vi ".NET Object Stream Writer.vi"(8 "error in (no error)":errorcluster, 9 "G Object":variant, 11 "TwinCAT ADS in":refnum<class "TwinCAT ADS.lvclass">) -> (0 "error out":errorcluster, 1 ".NET Object Stream":refnum<k24>[](array[refnum]), 2 ".NET Type Stream":refnum<k24>[](array[refnum]), 3 "TwinCAT ADS out":refnum<class "TwinCAT ADS.lvclass">)   [LabVIEW 2018, in "TwinCAT ADS.lvclass"]
uses:
  TwinCAT ADS.lvclass
  <vilib>/Utility/Data Type/NI_Data Type.lvlib
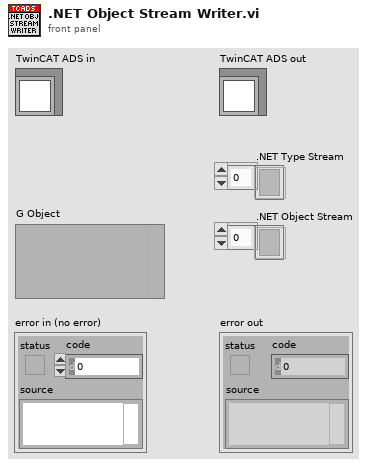
[diagram p1: front panel]
types:
  T1 = typedef "NI_Data Type.lvlib/Data Type.ctl" = enum8{"Invalid Type", "Void", "I8", "I16", "I32", "I64", "U8", "U16", "U32", "U64", "Single Float", "Double Float", "Extended Float", "Single Complex", "Double Complex", "Extended Complex", "Enum U8", "Enum U16", "Enum U32", "Enum U64", "Single Float With Unit", "Double Float With Unit", "Extended Float With Unit", "Single Complex with Unit", "Double Complex with Unit", "Extended Complex with Unit", "Boolean", "String", "Path", "Picture", "Tag", "Array", "Cluster", "Variant", "LV Variant", "Waveform", "Timestamp", "Digital Waveform", "Digital Data", "ExpressData", "Refnum", "External Data", "VI", "Poly VI", "LabVIEW Class Instance", "Fixed Point"}
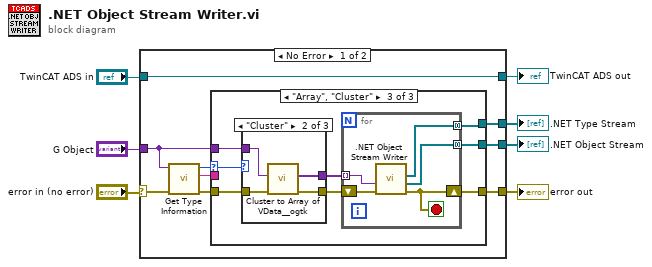
[diagram p0: block diagram]
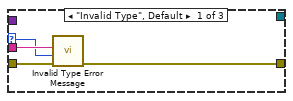
[diagram p2: hidden frame]
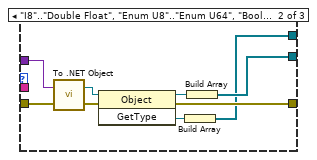
[diagram p3: hidden frame]
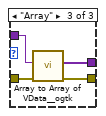
[diagram p5: hidden frame]
diagram:
  n1 = case shown="No Error" "error in (no error)" {
    selector: "error in (no error)" -> [w16 w53]
    tunnel: [w11 w53] -> w2
    tunnel: [w10 w52] -> w5
    tunnel: "TwinCAT ADS in" -> [w10 w52]
    tunnel: "G Object" -> [w14 _]
    tunnel: [w9 _] -> w3
    tunnel: [w8 _] -> w4
    frame No Error {
      n2 = call <vilib>:"Get Type Information.vi"("error in (no error)"=w16, "Variant"=w14) -> ("error out"=w13:errorcluster, "Name"=w12:string, "Type"=w15:T1)  [unwired: 5 in, 2 out]
      n3 = case shown="\"Array\", \"Cluster\"" w15 {
        selector: w15 -> [w18 _ w33]
        tunnel: w14 -> [_ w25 w36]
        tunnel: w13 -> [w20 w27 w37]
        tunnel: w12 -> [w19 _ _]
        tunnel: [w17 w26 w32] -> w11
        tunnel: [_ w23 w30] -> w9
        tunnel: [_ w21 w31] -> w8
        frame "Invalid Type", Default {
          n4 = call "Invalid Type Error Message.vi"("error in (no error)"=w20, "Type"=w18, "Name"=w19) -> ("error out"=w17:errorcluster)  [unwired: 7 in, 1 out]
        }
        frame "I8".."Double Float", "Enum U8".."Enum U64", "Boolean", "String" {
          n5 = call <vilib>:"To .NET Object.vi"("error in (no error)"=w27, "anything"=w25) -> ("error out"=w29:errorcluster, ".NET object"=w28:refnum<k24>)
          n6 = invoke class="Object" method="GetType"(reference=w28, error in=w29) -> (reference out=w24:refnum<k24>, error out=w26:errorcluster, "GetType"=w22:refnum<k24>)  [unwired: 1 in]
          n7 = Build Array(w22) -> (w21:refnum<k24>[])
          n8 = Build Array(w24) -> (w23:refnum<k24>[])
        }
        frame "Array", "Cluster" {
          n9 = case shown="\"Cluster\"" w33 {
            tunnel: w37 -> [w38 w42 w46]
            tunnel: w36 -> [_ w41 w44]
            tunnel: [w38 w40 w45] -> w35
            tunnel: [_ w39 w43] -> w34
            frame "Invalid Type", Default {
            }
            frame "Cluster" {
              n10 = call <userlib>:"Cluster to Array of VData__ogtk.vi"("error in (no error)"=w42, "Cluster"=w41) -> ("error out"=w40:errorcluster, "Array of VData"=w39:variant[])  [unwired: 8 in]
            }
            frame "Array" {
              n11 = call <userlib>:"Array to Array of VData__ogtk.vi"("error in (no error)"=w46, "MultiD Array"=w44) -> ("error out"=w45:errorcluster, "1D Array of Variants"=w43:variant[])  [unwired: 8 in]
            }
          }
          n12 = for {
            tunnel: w34 -> [w50] mode=indexing
            shift-right: [w49] -> w32
            shift-left: w35 -> [w51]
            tunnel: [w47] -> w31 mode=concatenating
            tunnel: [w48] -> w30 mode=concatenating
            stop <- w49 stop-if-true
            n13 = call ".NET Object Stream Writer.vi"("error in (no error)"=w51, "G Object"=w50) -> ("error out"=w49:errorcluster, ".NET Object Stream"=w48:refnum<k24>[], ".NET Type Stream"=w47:refnum<k24>[])  [unwired: 6 in, 1 out]
          }
        }
      }
    }
    frame Error {
    }
  }
  "error out" <- w2
  "TwinCAT ADS out" <- w5
  ".NET Type Stream" <- w4
  ".NET Object Stream" <- w3
